vi "Data File Processing UI Convert Message to String.vi"(7 "msg in":T1) -> (8 "msg":string)   [LabVIEW 2012]
uses:
  Data File Processing UI Message Define.ctl
  Data File Processing UI Message Type Define.ctl
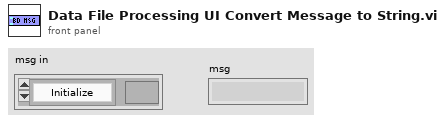
[diagram p1: front panel]
types:
  T1 = typedef "Data File Processing UI Message Define.ctl" = cluster{"data":variant, "type":T2}
  T2 = typedef "Data File Processing UI Message Type Define.ctl" = enum32{"Initialize", "SleepThread", "ErrorHandler", "NoEvent", "PreExit", "Exit", "----Action----", "OpenFile", "ReadAllCompute", "SaveFile", "RedrawGraph", "SelectChannel"}
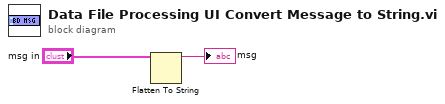
[diagram p0: block diagram]
diagram:
  n1 = Flatten To String(anything="msg in") -> (data string=→"msg":string)  [unwired: 3 in, 2 out]
